vi "_rszvl Default Instrument Setup.vi"(0 "VISA resource name":refnum<visa-resource-name>, 11 "error in (no error)":errorcluster) -> (4 "VISA resource name out":refnum<visa-resource-name>, 15 "error out":errorcluster)   [LabVIEW 2014]
doc: "This Utility VI sends a default command string to the instrument whenever a new VISA session is opened, or the instrument is reset. This VI is intended to be used as a subVI for the Initialize.vi and Reset VI. Altering this VI could cause these two VI's to operate incorrectly."
uses:
  rszvl_rsidr_core.lvlib
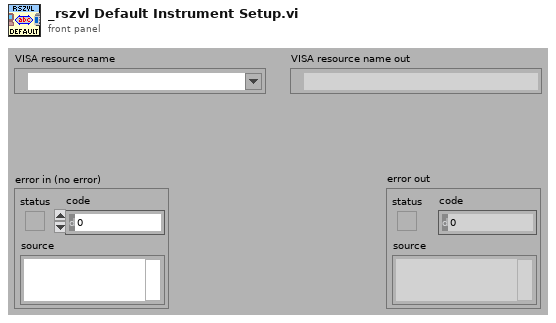
[diagram p1: front panel]
types:
  T1 = typedef "rszvl_rsidr_core.lvlib/type_Session_Data.ctl" = cluster{"Instr type":string, "Instr type for err. msg.":string, "Installed Options":string[], "OPC Timeout":i32, "Query Instrument Status":bool, "Check Range":bool, "Check Options":bool, "Add LF to Write":bool, "Simulate":bool, "Logging":bool, "Logging params":variant, "Interface Type":enum16{"Unknown", "GPIB", "VXI", "GPIB_VXI", "ASRL", "PXI", "TCPIP", "USB", "SOCKET"}, "Fast Sweep":i32, "AdditionalFlags":i32, "WaitBeforeWrite":i32, "WaitBeforeRead":i32, "BinDataChunkSize":i64}
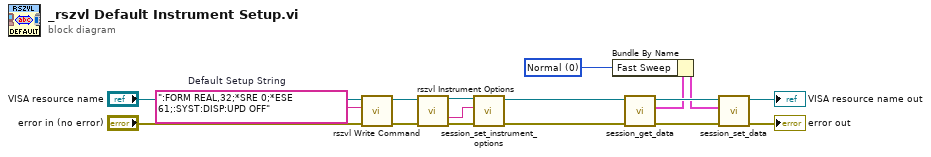
[diagram p0: block diagram]
diagram:
  w14 = 0 items=["Normal", "Fast"] ("Fast Sweep")
  w1 = ":FORM REAL,32;*SRE 0;*ESE 61;:SYST:DISP:UPD OFF"  # Default Setup String
  n1 = call "rszvl Write Command.vi"("error in (no error)"="error in (no error)", "Command"=w1, "VISA resource name"="VISA resource name") -> ("error out"=w17:errorcluster, "VISA resource name out"=w3:refnum<visa-resource-name>)  [unwired: 7 in]
  n2 = call "rszvl Instrument Options.vi"("VISA resource name"=w3, "error in (no error)"=w17) -> ("VISA resource name out"=w2:refnum<visa-resource-name>, "Options List"=w4:string, "error out"=w13:errorcluster)  [unwired: 11 in]
  n3 = call "session_set_instrument_options.vi"("error in"=w13, "Options string"=w4, "VISA resource name"=w2) -> ("error out"=w12:errorcluster, "VISA resource name out"=w11:refnum<visa-resource-name>)  [unwired: 7 in]
  n4 = call "session_get_data.vi"("error in"=w12, "VISA resource name"=w11) -> ("error out"=w10:errorcluster, "Session User Data out"=w6:T1, "VISA resource name out"=w9:refnum<visa-resource-name>)  [unwired: 7 in]
  n5 = Bundle By Name(cluster=w6, "Fast Sweep"=w14) -> (w5:T1)
  n6 = call "session_set_data.vi"("error in"=w10, "Session User Data in"=w5, "VISA resource name"=w9) -> ("error out"=→"error out":errorcluster, "VISA resource name out"=→"VISA resource name out":refnum<visa-resource-name>)  [unwired: 7 in]
